vi "Test - LabVIEW Object to VCluster.vi"(8 "error in":errorcluster) -> (0 "error out":errorcluster, 2 "pass?":bool)   [LabVIEW 2020, in "test_openg_array.lvlib"]
uses:
  test_openg_array.lvlib
  LVOOP Data/Class 1/Class 1.lvclass
  source/library/openg_variant.lvlib
  <vilib>/addons/_JKI Toolkits/Caraya/classes/Test/Test.lvclass
  <vilib>/addons/_JKI Toolkits/Caraya/classes/Assert/Assert.lvclass
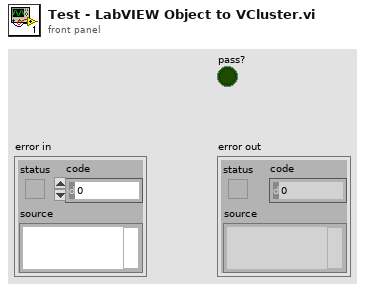
[diagram p1: front panel]
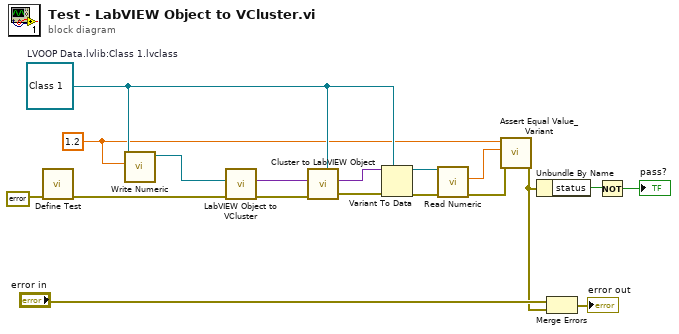
[diagram p0: block diagram]
diagram:
  w10 = 1.2 ("Numeric")
  w11 = refnum<class "Class 1.lvclass"> refnum  # LVOOP Data.lvlib:Class 1.lvclass
  n1 = call <vilib>:"Define Test.vi"("error in (no error)"=errorcluster {"status"=FALSE, "code"=0, "source"=""} ("error constant")) -> ("error out"=w6:errorcluster)  [unwired: 9 in, 1 out]
  n2 = call "Write Numeric.vi"("Numeric"=w10, "Class 1 in"=w11) -> ("Class 1 out"=w16:refnum<class "Class 1.lvclass">)  [unwired: 9 in]
  n3 = call "LabVIEW Object to VCluster.vi"("error in (no error)"=w6, "LabVIEW Object"=w16) -> ("error out"=w12:errorcluster, "VCluster"=w18:variant)  [unwired: 8 in]
  n4 = call "Cluster to LabVIEW Object.vi"("VObject Type"=w11, "error in (no error)"=w12, "VCluster"=w18) -> ("error out"=w13:errorcluster, "VObject out"=w17:variant)  [unwired: 7 in]
  n5 = Variant To Data(error in=w13, type=w11, Variant=w17) -> (data=w15:refnum<class "Class 1.lvclass">, error out=w14:errorcluster)
  n6 = call "Read Numeric.vi"("error in (no error)"=w14, "Class 1 in"=w15) -> ("error out"=w8:errorcluster, "Numeric"=w9:dbl)  [unwired: 7 in, 1 out]
  n7 = call <vilib>:"Assert Equal Value_Variant.vi"("error in (no error)"=w8, "Y"=w9, "X"=w10) -> ("error out"=w3:errorcluster)  [unwired: 7 in, 1 out]
  n8 = Unbundle By Name(w3) -> ("status"=w2:bool)
  n9 = Merge Errors("error in", w3) -> (→"error out":errorcluster)
  n10 = Not(x=w2) -> (.not. x?=→"pass?":bool)
